vi "KEI_Temperature.vi"(3 "error in":errorcluster, 4 "Language":T1, 5 "tempList":string="201", 6 "GPIB In":refnum<visa-resource-name>="GPIB0::16::INSTR") -> (0 "error out":errorcluster, 1 "Message":string, 2 "temprature":dbl)   [LabVIEW 2015]
uses:
  CustomControl/Lang_Control.ctl
  <instrlib>/Keithley 27XX/Public/Configure/Measurement Specific/Configure FRTD.vi
  <instrlib>/Keithley 27XX/Public/Data/Read Single Point.vi
  <instrlib>/Keithley 27XX/Keithley 27XX.lvlib
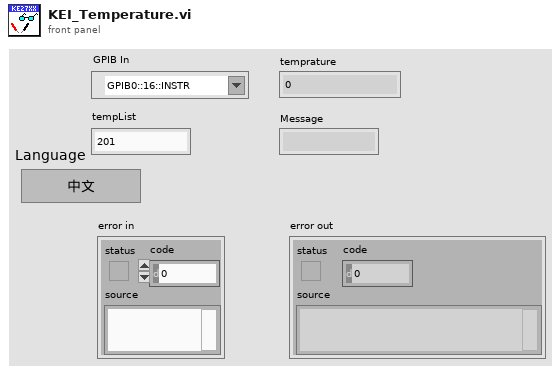
[diagram p1: front panel]
types:
  T1 = typedef "Lang_Control.ctl" = enum16{"中文", "English"}
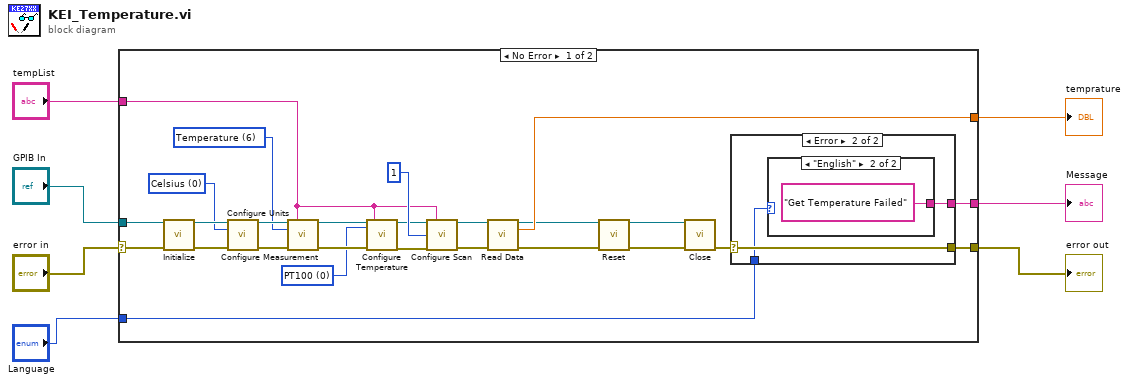
[diagram p0: block diagram]
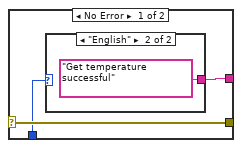
[diagram p2: hidden frame]
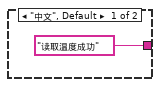
[diagram p3: hidden frame]
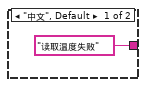
[diagram p4: hidden frame]
diagram:
  n1 = case shown="No Error" "error in" {
    selector: "error in" -> [w16 w44]
    tunnel: "tempList" -> [w19 _]
    tunnel: "GPIB In" -> [w18 _]
    tunnel: [w17 _] -> w5
    tunnel: [w14 w44] -> w4
    tunnel: [w13 _] -> w2
    tunnel: "Language" -> [w12 _]
    frame No Error {
      w25 = u16 0 items=["PT100", "D100", "F100", "PT3916", "PT385", "USER"] ("FRTD Type (0: PT100)")
      w28 = u16 6 items=["DC Voltage", "AC Voltage", "DC Current", "AC Current", "Resistance", "Four-Wire Resistance", "Temperature", "Frequency", "Period", "Continuity"] ("Function (0: DC Voltage)")
      w29 = u16 0 items=["Celsius", "Fahrenheit", "Kelvins"] ("Temperature (0: Celsius)")
      n2 = call <instrlib>:"Initialize.vi"("VISA resource name"=w18, "error in (no error)"=w16) -> ("VISA resource name out"=w33:refnum<visa-resource-name>, "error out"=w32:errorcluster)  [unwired: 12 in]
      n3 = call <instrlib>:"Configure Units.vi"("VISA resource name"=w33, "Temperature (0: Celsius)"=w29, "error in (no error)"=w32) -> ("VISA resource name out"=w31:refnum<visa-resource-name>, "error out"=w30:errorcluster)  [unwired: 11 in]
      n4 = call <instrlib>:"Configure Measurement.vi"("VISA resource name"=w31, "Scan List (Empty)"=w19, "Function (0: DC Voltage)"=w28, "error in (no error)"=w30) -> ("VISA resource name out"=w27:refnum<visa-resource-name>, "error out"=w26:errorcluster)  [unwired: 10 in]
      n5 = call-poly <instrlib>:"Configure Temperature.vi"("VISA resource name"=w27, "FRTD Type (0: PT100)"=w25, "error in (no error)"=w26, "Scan List (Empty)"=w19) -> ("VISA resource name out"=w23:refnum<visa-resource-name>, "error out"=w22:errorcluster)  [unwired: 14 in]
      n6 = call <instrlib>:"Configure Scan.vi"("VISA resource name"=w23, "Channel List (101:110)"=w19, "Sample Count (100)"=1, "error in (no error)"=w22) -> ("VISA resource name out"=w20:refnum<visa-resource-name>, "error out"=w21:errorcluster)  [unwired: 10 in]
      n7 = call-poly <instrlib>:"Read Data.vi"("VISA resource name"=w20, "error in (no error)"=w21) -> ("VISA resource name out"=w11:refnum<visa-resource-name>, "Measurement Data"=w17:dbl, "error out"=w9:errorcluster)  [unwired: 11 in]
      n8 = call <instrlib>:"Reset.vi"("VISA resource name"=w11, "error in (no error)"=w9) -> ("VISA resource name out"=w10:refnum<visa-resource-name>, "error out"=w8:errorcluster)  [unwired: 12 in]
      n9 = call <instrlib>:"Close.vi"("VISA resource name"=w10, "error in (no error)"=w8) -> ("error out"=w15:errorcluster)  [unwired: 13 in]
      n10 = case shown="Error" w15 {
        selector: w15 -> [w35 w40]
        tunnel: [w36 w41] -> w13
        tunnel: [w35 w40] -> w14
        tunnel: w12 -> [w34 w39]
        frame No Error {
          n11 = case shown="\"English\"" w34 {
            tunnel: ["读取温度成功" "Get temperature successful"] -> w36
            frame "中文", Default {
            }
            frame "English" {
            }
          }
        }
        frame Error {
          n12 = case shown="\"English\"" w39 {
            tunnel: ["读取温度失败" "Get Temperature Failed"] -> w41
            frame "中文", Default {
            }
            frame "English" {
            }
          }
        }
      }
    }
    frame Error {
    }
  }
  "error out" <- w4
  "temprature" <- w5
  "Message" <- w2
